vi "读取解析.vi"(10 "读取data":u8[](array[numeric]), 11 "格式字符串":string) -> (3 "输出字符串":string)   [LabVIEW 2016]
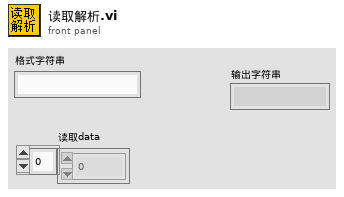
[diagram p1: front panel]
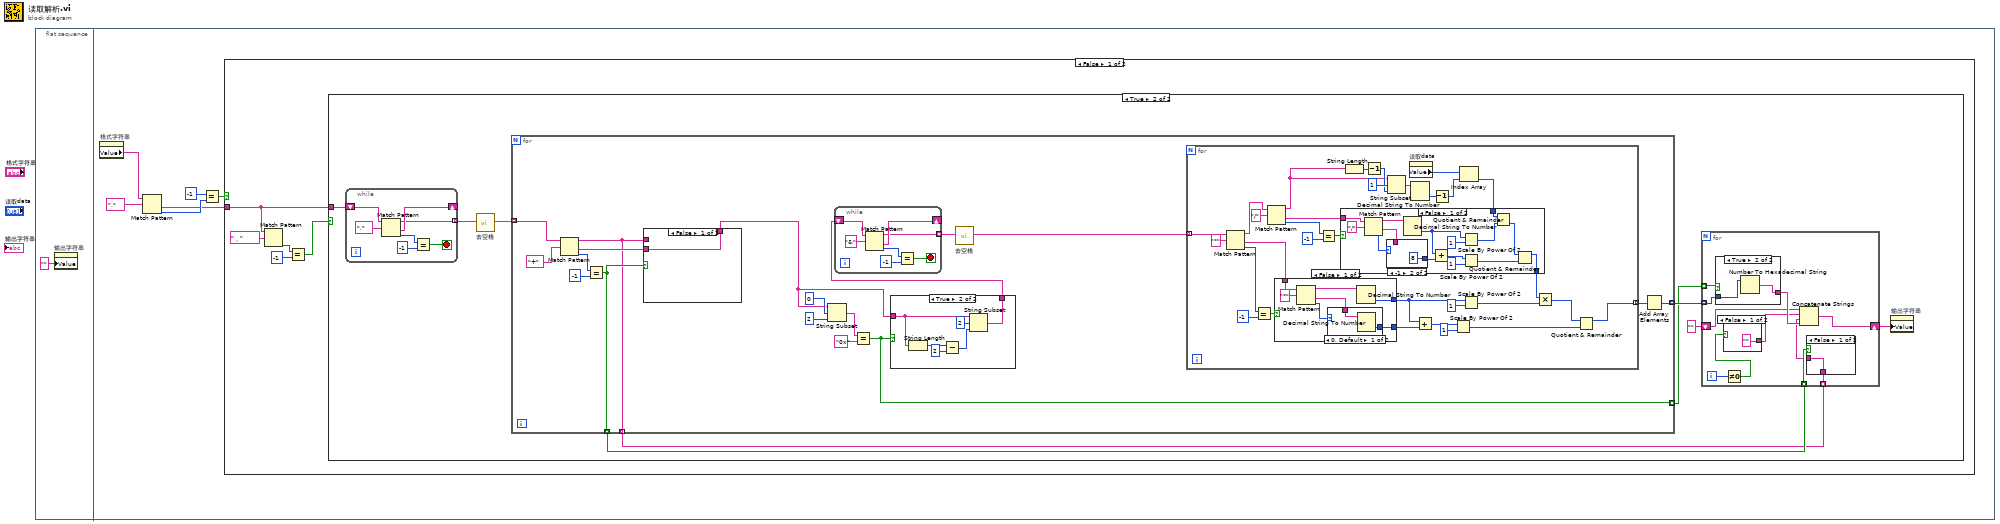
[diagram p0: block diagram]
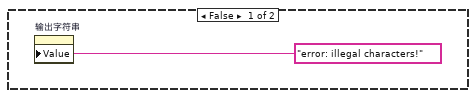
[diagram p2: hidden frame]
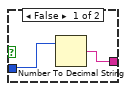
[diagram p3: hidden frame]
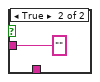
[diagram p4: hidden frame]
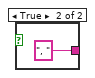
[diagram p5: hidden frame]
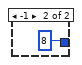
[diagram p8: hidden frame]
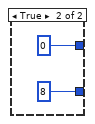
[diagram p9: hidden frame]
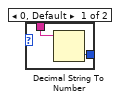
[diagram p10: hidden frame]
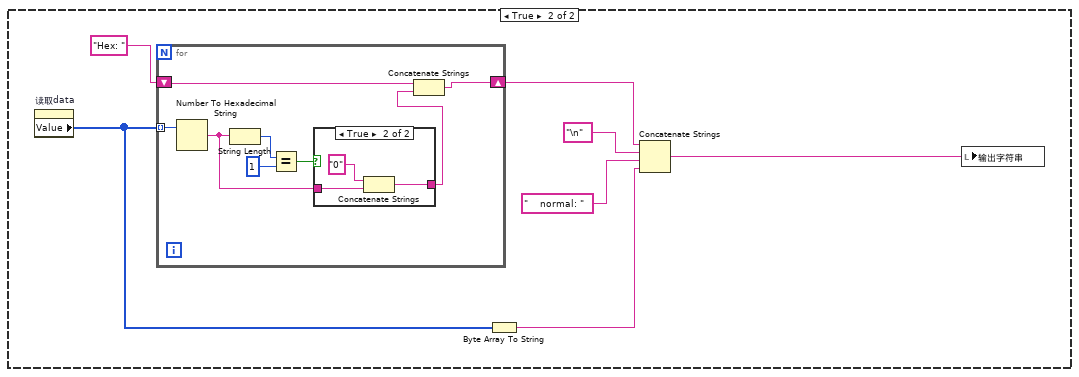
[diagram p12: hidden frame]
diagram:
  n1 = flat-sequence {
    frame #0 {
      n2 = property on="输出字符串" class="Str"("Value"="" ("输出字符串")) -> ()  [unwired: 2 in, 2 out]
    }
    frame #1 {
      n3 = property on="格式字符串" class="Str"() -> ("Value"=w3:string)  [unwired: 2 in, 2 out]
      n4 = Match Pattern(string=w3, regular expression=",") -> (after substring=w4:string, offset past match=w6:i32)  [unwired: 1 in, 2 out]
      n5 = Equal?(x=-1, y=w6) -> (x = y?=w7:bool)
      n6 = case shown="False" w7 {
        tunnel: w4 -> [w12 _]
        frame False {
          n7 = Match Pattern(string=w12, regular expression="，") -> (offset past match=w10:i32)  [unwired: 1 in, 3 out]
          n8 = Equal?(x=w10, y=-1) -> (x = y?=w8:bool)
          n9 = case shown="True" w8 {
            tunnel: w12 -> [_ w22]
            frame False {
              n10 = property on="输出字符串" class="Str"("Value"="error: illegal characters!" ("输出字符串")) -> ()  [unwired: 2 in, 2 out]
            }
            frame True {
              n11 = while {
                shift-right: [w143] -> _
                shift-left: w22 -> [w144]
                tunnel: [w142] -> w21 mode=indexing
                stop <- w138 stop-if-true
                n12 = Match Pattern(string=w144, regular expression=",") -> (before substring=w142:string, after substring=w143:string, offset past match=w140:i32)  [unwired: 1 in, 1 out]
                n13 = Equal?(x=w140, y=-1) -> (x = y?=w138:bool)
              }
              n14 = call "去空格.vi"("Array"=w21) -> ("Array out"=w20:string[])  [unwired: 9 in, 1 out]
              n15 = for {
                tunnel: w20 -> [w51] mode=indexing
                tunnel: [w56] -> w19 mode=indexing
                tunnel: [w50] -> w16 mode=indexing
                tunnel: [w49] -> w15 mode=indexing
                tunnel: [w42] -> w14 mode=indexing
                n16 = Match Pattern(string=w51, regular expression="+") -> (before substring=w49:string, after substring=w52:string, offset past match=w54:i32)  [unwired: 1 in, 1 out]
                n17 = Equal?(x=w54, y=-1) -> (x = y?=w50:bool)
                n18 = case shown="False" w50 {
                  tunnel: w49 -> [_ w68]
                  tunnel: w52 -> [w67 _]
                  tunnel: [w67 w68] -> w44
                  frame False {
                  }
                  frame True {
                  }
                }
                n19 = String Subset(string=w44, offset (0)=0, length (rest)=2 ("length (rest)")) -> (substring=w48:string)
                n20 = Equal?(x=w48, y="0x") -> (x = y?=w42:bool)
                n21 = case shown="True" w42 {
                  tunnel: w44 -> [w60 w66]
                  tunnel: [w60 w61] -> w43
                  frame False {
                  }
                  frame True {
                    n22 = String Length(string=w66) -> (length=w64:i32)
                    n23 = Subtract(x=w64, y=2) -> (x-y=w63:i32)
                    n24 = String Subset(string=w66, offset (0)=2, length (rest)=w63) -> (substring=w61:string)
                  }
                }
                n25 = while {
                  shift-right: [w136] -> _
                  shift-left: w43 -> [w137]
                  tunnel: [w135] -> w59 mode=indexing
                  stop <- w131 stop-if-true
                  n26 = Match Pattern(string=w137, regular expression="&") -> (before substring=w135:string, after substring=w136:string, offset past match=w133:i32)  [unwired: 1 in, 1 out]
                  n27 = Equal?(x=w133, y=-1) -> (x = y?=w131:bool)
                }
                n28 = call "去空格.vi"("Array"=w59) -> ("Array out"=w58:string[])  [unwired: 9 in, 1 out]
                n29 = for {
                  tunnel: w58 -> [w79] mode=indexing
                  tunnel: [w72] -> w57 mode=indexing
                  n30 = Match Pattern(string=w79, regular expression="*") -> (before substring=w96:string, after substring=w98:string, offset past match=w70:i32)  [unwired: 1 in, 1 out]
                  n31 = Equal?(x=w70, y=-1) -> (x = y?=w71:bool)
                  n32 = Match Pattern(string=w96, regular expression="/") -> (before substring=w91:string, after substring=w95:string, offset past match=w81:i32)  [unwired: 1 in, 1 out]
                  n33 = case shown="False" w71 {
                    tunnel: w98 -> [w105 _]
                    tunnel: [w102 0] -> w77
                    tunnel: [w101 8] -> w76
                    frame False {
                      n34 = Match Pattern(string=w105, regular expression="*") -> (before substring=w104:string, after substring=w103:string, offset past match=w100:i32)  [unwired: 1 in, 1 out]
                      n35 = case shown="0, Default" w100 {
                        tunnel: w103 -> [w108 _]
                        tunnel: [w107 8] -> w101
                        frame 0, Default {
                          n36 = Decimal String To Number(string=w108) -> (number=w107:i32)  [unwired: 2 in, 1 out]
                        }
                        frame -1 {
                        }
                      }
                      n37 = Decimal String To Number(string=w104) -> (number=w102:i32)  [unwired: 2 in, 1 out]
                    }
                    frame True {
                    }
                  }
                  n38 = Equal?(x=w81, y=-1) -> (x = y?=w82:bool)
                  n39 = String Length(string=w91) -> (length=w93:i32)
                  n40 = Decrement(x=w93) -> (x-1=w92:i32)
                  n41 = String Subset(string=w91, offset (0)=u64 1, length (rest)=w92) -> (substring=w90:string)
                  n42 = property on="读取data" class="Arr (strict)"() -> ("Value"=w89:u8[])  [unwired: 2 in, 2 out]
                  n43 = Decimal String To Number(string=w90) -> (number=w88:i32)  [unwired: 2 in, 1 out]
                  n44 = Add(x=w77, y=w76) -> (x+y=w75:i32)
                  n45 = Decrement(x=w88) -> (x-1=w83:i32)
                  n46 = Scale By Power Of 2(n=w75, x=u32 1) -> (x*2^n=w73:u32)
                  n47 = Index Array(array=w89, index=w83) -> (element=w87:u8)
                  n48 = case shown="False" w82 {
                    tunnel: w95 -> [w125 _]
                    tunnel: w87 -> [w119 w130]
                    tunnel: [w116 w130] -> w84
                    frame False {
                      n49 = Match Pattern(string=w125, regular expression="/") -> (before substring=w124:string, after substring=w123:string, offset past match=w112:i32)  [unwired: 1 in, 1 out]
                      n50 = case shown="-1" w112 {
                        tunnel: w123 -> [w128 _]
                        tunnel: [w127 8] -> w115
                        frame 0, Default {
                          n51 = Decimal String To Number(string=w128) -> (number=w127:i32)  [unwired: 2 in, 1 out]
                        }
                        frame -1 {
                        }
                      }
                      n52 = Decimal String To Number(string=w124) -> (number=w114:i32)  [unwired: 2 in, 1 out]
                      n53 = Add(x=w114, y=w115) -> (x+y=w113:i32)
                      n54 = Scale By Power Of 2(n=w114, x=u32 1) -> (x*2^n=w120:u32)
                      n55 = Scale By Power Of 2(n=w113, x=u32 1) -> (x*2^n=w117:u32)
                      n56 = Quotient & Remainder(x=w119, y=w120) -> (floor(x/y)=w118:u32)  [unwired: 1 out]
                      n57 = Quotient & Remainder(x=w118, y=w117) -> (x-y*floor(x/y)=w116:u32)  [unwired: 1 out]
                    }
                    frame True {
                    }
                  }
                  n58 = Scale By Power Of 2(n=w77, x=u32 1) -> (x*2^n=w85:u32)
                  n59 = Multiply(x=w84, y=w85) -> (x*y=w74:u32)
                  n60 = Quotient & Remainder(x=w74, y=w73) -> (x-y*floor(x/y)=w72:u32)  [unwired: 1 out]
                }
                n61 = Add Array Elements(numeric array=w57) -> (sum=w56:u32)
              }
              n62 = for {
                tunnel: w19 -> [w33] mode=indexing
                shift-right: [w32] -> w17
                shift-left: "" -> [w28]
                tunnel: w16 -> [w26] mode=indexing
                tunnel: w15 -> [w25] mode=indexing
                tunnel: w14 -> [w23] mode=indexing
                i -> [w30]
                n63 = case shown="True" w23 {
                  tunnel: w33 -> [w35 w37]
                  tunnel: [w34 w36] -> w31
                  frame False {
                    n64 = Number To Decimal String(number=w35) -> (decimal integer string=w34:string)  [unwired: 1 in]
                  }
                  frame True {
                    n65 = Number To Hexadecimal String(2:w37) -> (0:w36:string)  [unwired: 1 in]
                  }
                }
                n66 = Not Equal To 0?(x=w30) -> (x != 0?=w29:bool)
                n67 = case shown="False" w29 {
                  tunnel: ["" ("string") ", " ("string")] -> w27
                  frame False {
                  }
                  frame True {
                  }
                }
                n68 = case shown="False" w26 {
                  tunnel: w25 -> [w38 _]
                  tunnel: [w38 "" ("String")] -> w24
                  frame False {
                  }
                  frame True {
                  }
                }
                n69 = Concatenate Strings(w28, w27, w24, w31) -> (w32:string)
              }
              n70 = property on="输出字符串" class="Str"("Value"=w17) -> ()  [unwired: 2 in, 2 out]
            }
          }
        }
        frame True {
          n71 = property on="读取data" class="Arr (strict)"() -> ("Value"=w150:u8[])  [unwired: 2 in, 2 out]
          n72 = for {
            tunnel: w150 -> [w159] mode=indexing
            shift-right: [w152] -> w149
            shift-left: "Hex: " -> [w154]
            n73 = Number To Hexadecimal String(2:w159) -> (0:w155:string)  [unwired: 1 in]
            n74 = String Length(string=w155) -> (length=w158:i32)
            n75 = Equal?(x=w158, y=1) -> (x = y?=w156:bool)
            n76 = case shown="True" w156 {
              tunnel: w155 -> [w160 w163]
              tunnel: [w160 w161] -> w153
              frame False {
              }
              frame True {
                n77 = Concatenate Strings("0" ("string"), w163) -> (w161:string)
              }
            }
            n78 = Concatenate Strings(w154, w153) -> (w152:string)
          }
          n79 = Byte Array To String(unsigned byte array=w150) -> (string=w146:string)
          n80 = Concatenate Strings(w149, "\n" ("string"), "    normal: " ("string"), w146) -> (w145:string)
          n81 = local write "输出字符串"(w145) -> ()
        }
      }
    }
  }
